vi "Set Initialization Data - Settings.vi"(8 "error in":errorcluster, 11 "Debug Server in":refnum<class "Debug Server.lvclass">) -> (0 "error out":errorcluster, 3 "Debug Server out":refnum<class "Debug Server.lvclass">)   [LabVIEW 2017, in "Debug Server.lvclass"]
doc: "Sets the initialization data of a statically linked subWorker."
uses:
  Debug Server.lvclass
  Settings/Initialization Data.ctl
  Settings/Response Cases.ctl
  <vilib>/addons/_Workers/Library/Case Label.ctl
  Debug Server.lvclass/Debug Server.ctl
  Settings/Settings.lvclass
  C:/Program Files (x86)/National Instruments/LabVIEW 2017/vi.lib/addons/_Workers/Library/Classes/Worker/Worker.lvclass
  <vilib>/addons/_Workers/Library/Workers.lvlib
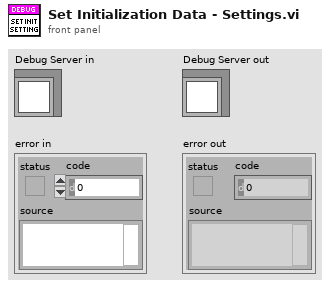
[diagram p1: front panel]
types:
  T1 = typedef "Settings.lvclass/Initialization Data.ctl" = cluster{"Response Cases":T2}
  T2 = typedef "Settings.lvclass/Response Cases.ctl" = cluster{"Configuration Data":T3, "Shutdown Data Written to File":T3}
  T3 = typedef "Workers.lvlib/Case Label.ctl" = string
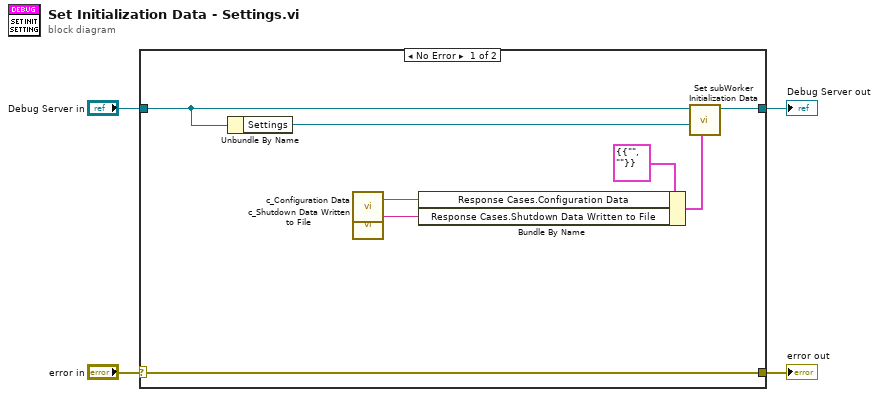
[diagram p0: block diagram]
diagram:
  n1 = case shown="No Error" "error in" {
    selector: "error in" -> [w12 w14]
    tunnel: [w12 w14] -> w3
    tunnel: [w10 w13] -> w2
    tunnel: "Debug Server in" -> [w9 w13]
    frame No Error {
      n2 = Unbundle By Name(w9) -> ("Settings"=w11:refnum<class "Settings.lvclass">)
      n3 = call "c_Configuration Data.vi"() -> ("Case Label"=w6:T3)  [unwired: 1 in]
      n4 = call "c_Shutdown Data Written to File.vi"() -> ("Case Label"=w5:T3)  [unwired: 1 in]
      n5 = Bundle By Name(cluster=T1 {"Response Cases"={"Configuration Data"="", "Shutdown Data Written to File"=""}} ("Initialization Data"), "Response Cases.Configuration Data"=w6, "Response Cases.Shutdown Data Written to File"=w5) -> (w8:T1)
      n6 = call-dynamic "Set subWorker Initialization Data.vi"("Initialization Data"=w8, "subWorker"=w11, "Worker"=w9) -> ("Worker out"=w10:refnum<class "Debug Server.lvclass">)  [unwired: 8 in]
    }
    frame Error {
    }
  }
  "error out" <- w3
  "Debug Server out" <- w2
